vi "query.vi"(2 "数据输入":string, 3 "连接ID":refnum<k5>) -> (0 "数据输出":string, 1 "连接ID输出":refnum<k5>)   [LabVIEW 2017]
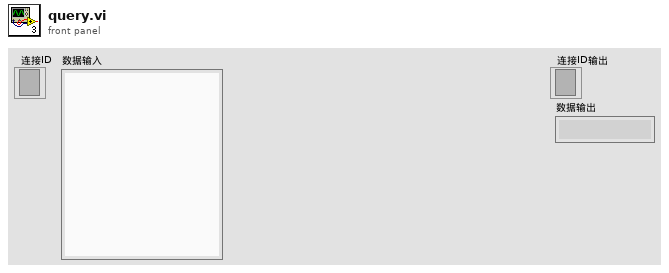
[diagram p1: front panel]
types:
  T1 = typedef "Semaphore RefNum" = refnum<k1>
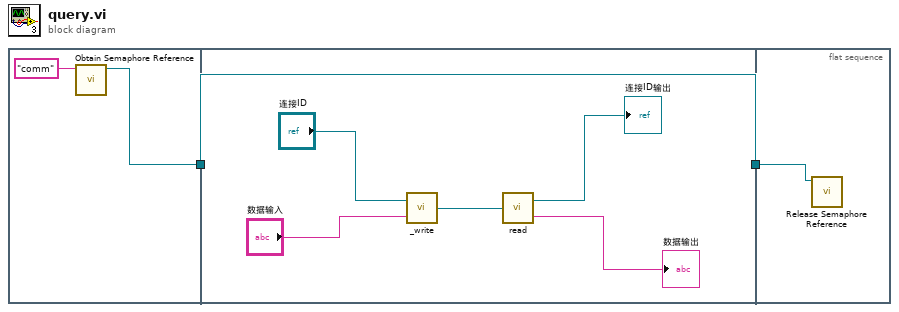
[diagram p0: block diagram]
diagram:
  n1 = flat-sequence {
    tunnel: [w4] -> w1
    tunnel: [w5] -> w2
    tunnel: w1 -> [w5]
    tunnel: w2 -> [w11]
    frame #0 {
      n2 = call <vilib>:"Obtain Semaphore Reference.vi"("name (unnamed)"="comm") -> ("semaphore"=w4:T1)  [unwired: 4 in, 2 out]
    }
    frame #1 {
      n3 = call "_write.vi"("数据输入"="数据输入", "连接ID"="连接ID") -> ("连接ID输出"=w10:refnum<k5>)
      n4 = call "read.vi"("连接ID"=w10) -> ("连接ID输出"=→"连接ID输出":refnum<k5>, "数据输出"=→"数据输出":string)
    }
    frame #2 {
      n5 = call <vilib>:"Release Semaphore Reference.vi"("semaphore"=w11) -> ()  [unwired: 9 in, 2 out]
    }
  }
